vi "GPIOs.vi"(8 "error in (no error)":errorcluster, 11 "I2C in":refnum<class "I2C.lvclass">) -> (0 "error out":errorcluster, 1 "SDA GPIO":T1, 2 "SCL GPIO":T1, 3 "I2C out":refnum<class "I2C.lvclass">)   [LabVIEW 2024, in "CTI.lvlib" / "I2C.lvclass"]
uses:
  I2C.lvclass
  GPIO Number.ctl
  I2C.lvclass/I2C.ctl
  CTI.lvlib
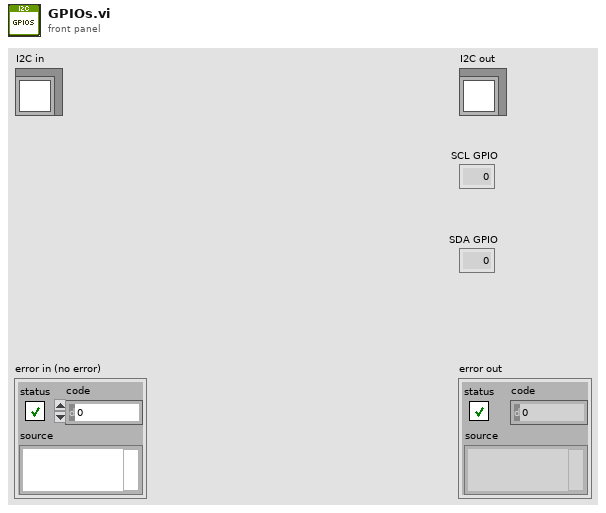
[diagram p1: front panel]
types:
  T1 = typedef "CTI.lvlib/GPIO Number.ctl" = i8
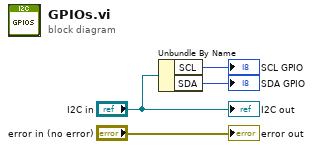
[diagram p0: block diagram]
diagram:
  n1 = Unbundle By Name("I2C in") -> ("SCL"=→"SCL GPIO":T1, "SDA"=→"SDA GPIO":T1)
  "error out" <- "error in (no error)"
  "I2C out" <- "I2C in"
